vi "Cargo Manip Control.vi"   [LabVIEW 2018]
uses:
  SubSystems/Cargo Intake/Cargo Intake Global.vi
  SubSystems/Controllers/Manipulator Controlller/Manipulator Controller Global.vi
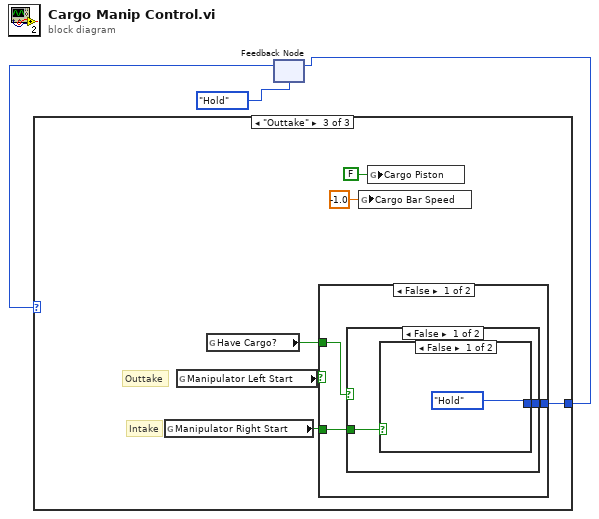
[diagram p0: block diagram]
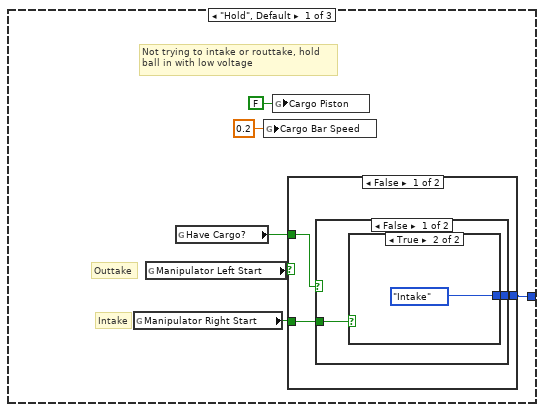
[diagram p2: hidden frame]
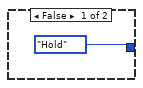
[diagram p3: hidden frame]
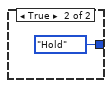
[diagram p4: hidden frame]
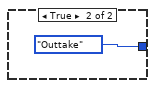
[diagram p5: hidden frame]
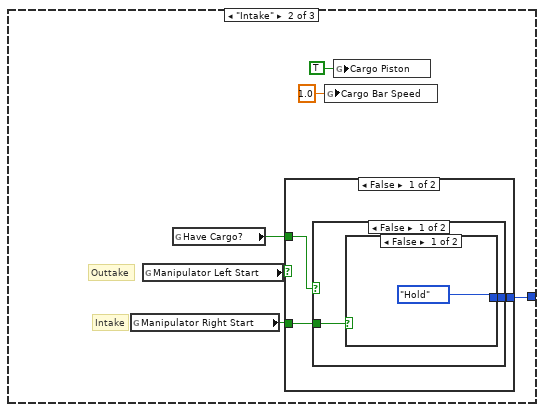
[diagram p6: hidden frame]
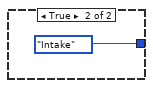
[diagram p7: hidden frame]
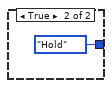
[diagram p8: hidden frame]
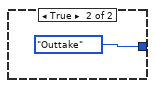
[diagram p9: hidden frame]
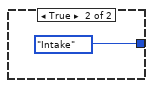
[diagram p10: hidden frame]
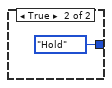
[diagram p11: hidden frame]
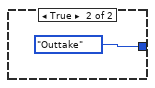
[diagram p12: hidden frame]
diagram:
  n1 = feedback #1(enum16{"Going Up", "Outtake", "Intake", "Hold"}."Hold") -> (w2:enum16{"Going Up", "Outtake", "Intake", "Hold"})
  n2 = case shown="\"Outtake\"" w2 {
    tunnel: [w4 w19 w34] -> w1
    frame "Hold", Default {
      # "Outtake"
      # "Intake"
      # "Not trying to intake or routtake, hold\nball in with low voltage"
      n3 = global read "Manipulator Controller Global.vi" "Manipulator Right Start"() -> (w7:bool)
      n4 = global read "Manipulator Controller Global.vi" "Manipulator Left Start"() -> (w6:bool)
      n5 = global read "Cargo Intake Global.vi" "Have Cargo?"() -> (w5:bool)
      n6 = global write "Cargo Intake Global.vi" "Cargo Bar Speed"(0.2 ("Cargo Bar Speed")) -> ()
      n7 = global write "Cargo Intake Global.vi" "Cargo Piston"(FALSE ("Cargo Piston")) -> ()
      n8 = case shown="False" w6 {
        tunnel: w7 -> [w12 _]
        tunnel: [w11 enum16{"Going Up", "Outtake", "Intake", "Hold"}."Outtake"] -> w4
        tunnel: w5 -> [w10 _]
        frame False {
          n9 = case shown="False" w10 {
            tunnel: w12 -> [w14 _]
            tunnel: [w13 enum16{"Going Up", "Outtake", "Intake", "Hold"}."Hold"] -> w11
            frame False {
              n10 = case shown="True" w14 {
                tunnel: [enum16{"Going Up", "Outtake", "Intake", "Hold"}."Hold" enum16{"Going Up", "Outtake", "Intake", "Hold"}."Intake"] -> w13
                frame False {
                }
                frame True {
                }
              }
            }
            frame True {
            }
          }
        }
        frame True {
        }
      }
    }
    frame "Intake" {
      # "Outtake"
      # "Intake"
      n11 = global read "Manipulator Controller Global.vi" "Manipulator Right Start"() -> (w24:bool)
      n12 = global read "Manipulator Controller Global.vi" "Manipulator Left Start"() -> (w23:bool)
      n13 = global read "Cargo Intake Global.vi" "Have Cargo?"() -> (w22:bool)
      n14 = case shown="False" w23 {
        tunnel: w24 -> [w27 _]
        tunnel: [w26 enum16{"Going Up", "Outtake", "Intake", "Hold"}."Outtake"] -> w19
        tunnel: w22 -> [w25 _]
        frame False {
          n15 = case shown="False" w25 {
            tunnel: w27 -> [w29 _]
            tunnel: [w28 enum16{"Going Up", "Outtake", "Intake", "Hold"}."Hold"] -> w26
            frame False {
              n16 = case shown="False" w29 {
                tunnel: [enum16{"Going Up", "Outtake", "Intake", "Hold"}."Hold" enum16{"Going Up", "Outtake", "Intake", "Hold"}."Intake"] -> w28
                frame False {
                }
                frame True {
                }
              }
            }
            frame True {
            }
          }
        }
        frame True {
        }
      }
      n17 = global write "Cargo Intake Global.vi" "Cargo Bar Speed"(1.0 ("Cargo Bar Speed")) -> ()
      n18 = global write "Cargo Intake Global.vi" "Cargo Piston"(TRUE ("Cargo Piston")) -> ()
    }
    frame "Outtake" {
      # "Outtake"
      # "Intake"
      n19 = global read "Manipulator Controller Global.vi" "Manipulator Right Start"() -> (w39:bool)
      n20 = global read "Manipulator Controller Global.vi" "Manipulator Left Start"() -> (w38:bool)
      n21 = global read "Cargo Intake Global.vi" "Have Cargo?"() -> (w37:bool)
      n22 = case shown="False" w38 {
        tunnel: w39 -> [w42 _]
        tunnel: [w41 enum16{"Going Up", "Outtake", "Intake", "Hold"}."Outtake"] -> w34
        tunnel: w37 -> [w40 _]
        frame False {
          n23 = case shown="False" w40 {
            tunnel: w42 -> [w44 _]
            tunnel: [w43 enum16{"Going Up", "Outtake", "Intake", "Hold"}."Hold"] -> w41
            frame False {
              n24 = case shown="False" w44 {
                tunnel: [enum16{"Going Up", "Outtake", "Intake", "Hold"}."Hold" enum16{"Going Up", "Outtake", "Intake", "Hold"}."Intake"] -> w43
                frame False {
                }
                frame True {
                }
              }
            }
            frame True {
            }
          }
        }
        frame True {
        }
      }
      n25 = global write "Cargo Intake Global.vi" "Cargo Bar Speed"(-1.0 ("Cargo Bar Speed")) -> ()
      n26 = global write "Cargo Intake Global.vi" "Cargo Piston"(FALSE ("Cargo Piston")) -> ()
    }
  }
  n27 = feedback-in #1(w1) -> ()
